vi "Condition Finish Create.vi"(4 "Actor Ref":refnum<vi>, 5 "Alias":string, 6 "Creator Attributes":refnum<class "Attributes.lvclass">, 7 "Unified Msg Set":T1, 10 "Queue of Self Attributes":refnum<queue>, 11 "Actor in":refnum<class "Actor.lvclass">) -> (0 "Error out":errorcluster, 3 "Actor out":refnum<class "Actor.lvclass">)   [LabVIEW 2020, in "jettl.lvlib" / "Actor.lvlib" / "Actor.lvclass"]
uses:
  Actor.lvclass
  Attributes/Attributes/Attributes.lvclass
  Msg Set.ctl
  Msg/Msg.lvclass
  Actor.lvlib
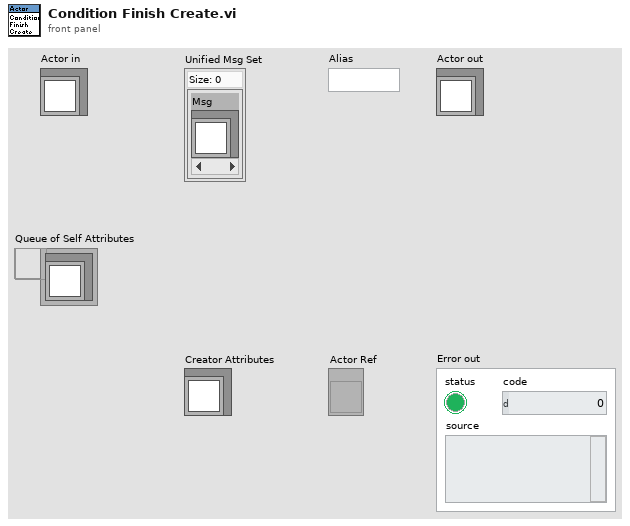
[diagram p1: front panel]
types:
  T1 = typedef "jettl.lvlib/Actor.lvlib/Msg Set.ctl" = set{refnum<class "Msg.lvclass">}
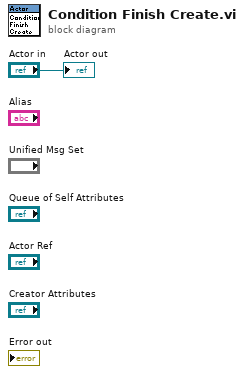
[diagram p0: block diagram]
diagram:
  "Actor out" <- "Actor in"
